vi "1.1)Comandos trigger.vi"() -> ()   [LabVIEW 2014]
panel:
  out "Comando a enviar":string
  in  "?":bool
  out "Comando final":string
  in  "Force":bool
  out "Comandos flanco":string
  out "Comandos pulso":string
  out "Comandos Video":string
  in  "State":bool
  in  "Frecuency":bool
  in  "Mode":u16(ring) items=["Auto", "Normal"]
  in  "Holdoff":dbl(knob) scale=5e-07..10.0
  in  "Nivel":dbl(knob) scale=-20.0..20.0
  out "Tipo de trigger":string
  in  "Opciones de Trigger":enum32{"Flanco", "Video", "Pulso"}(tab)
  in  "Canal":u16(ring) items=["Canal 1", "Canal 2"]
  in  "Slope":u16(ring) items=["Fall", "Rise"]
  in  "Acoplamiento":u16(ring) items=["AC", "DC", "Sin altas frecuencias DC", "Sin bajas frecuencias AC", "Baja sensibilidad DC"]
  in  "Sync":u16(ring) items=["Field", "Line", "Odd", "Even", "LineNum"]
  in  "Polarity":u16(ring) items=["Inverted", "Normal"]
  in  "Lines":dbl(knob) scale=0.0..525.0
  in  "Standard":u16(ring) items=["NTSC", "PAL"]
  in  "Canal":u16(ring) items=["Canal 1", "Canal 2"]
  in  "Width":dbl(knob) scale=3.3e-08..10.0
  in  "When":u16(ring) items=["Equal", "NotEqual", "Inside", "Outside"]
  in  "Polarity":u16(ring) items=["Positivo", "Negativo"]
  in  "Ancho":u16(ring) items=["Polarity", "When", "Width"]
  in  "Canal":u16(ring) items=["Canal 1", "Canal 2"]
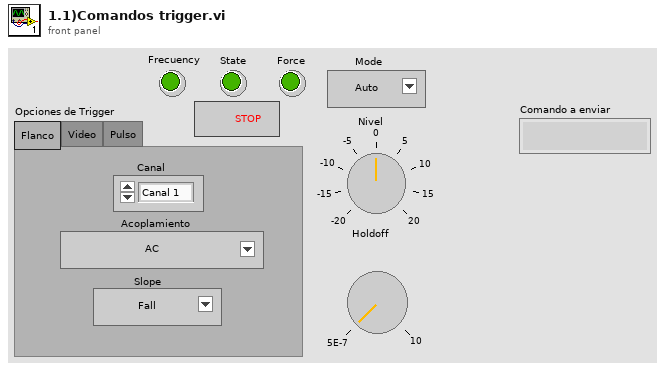
[diagram p1: front panel]
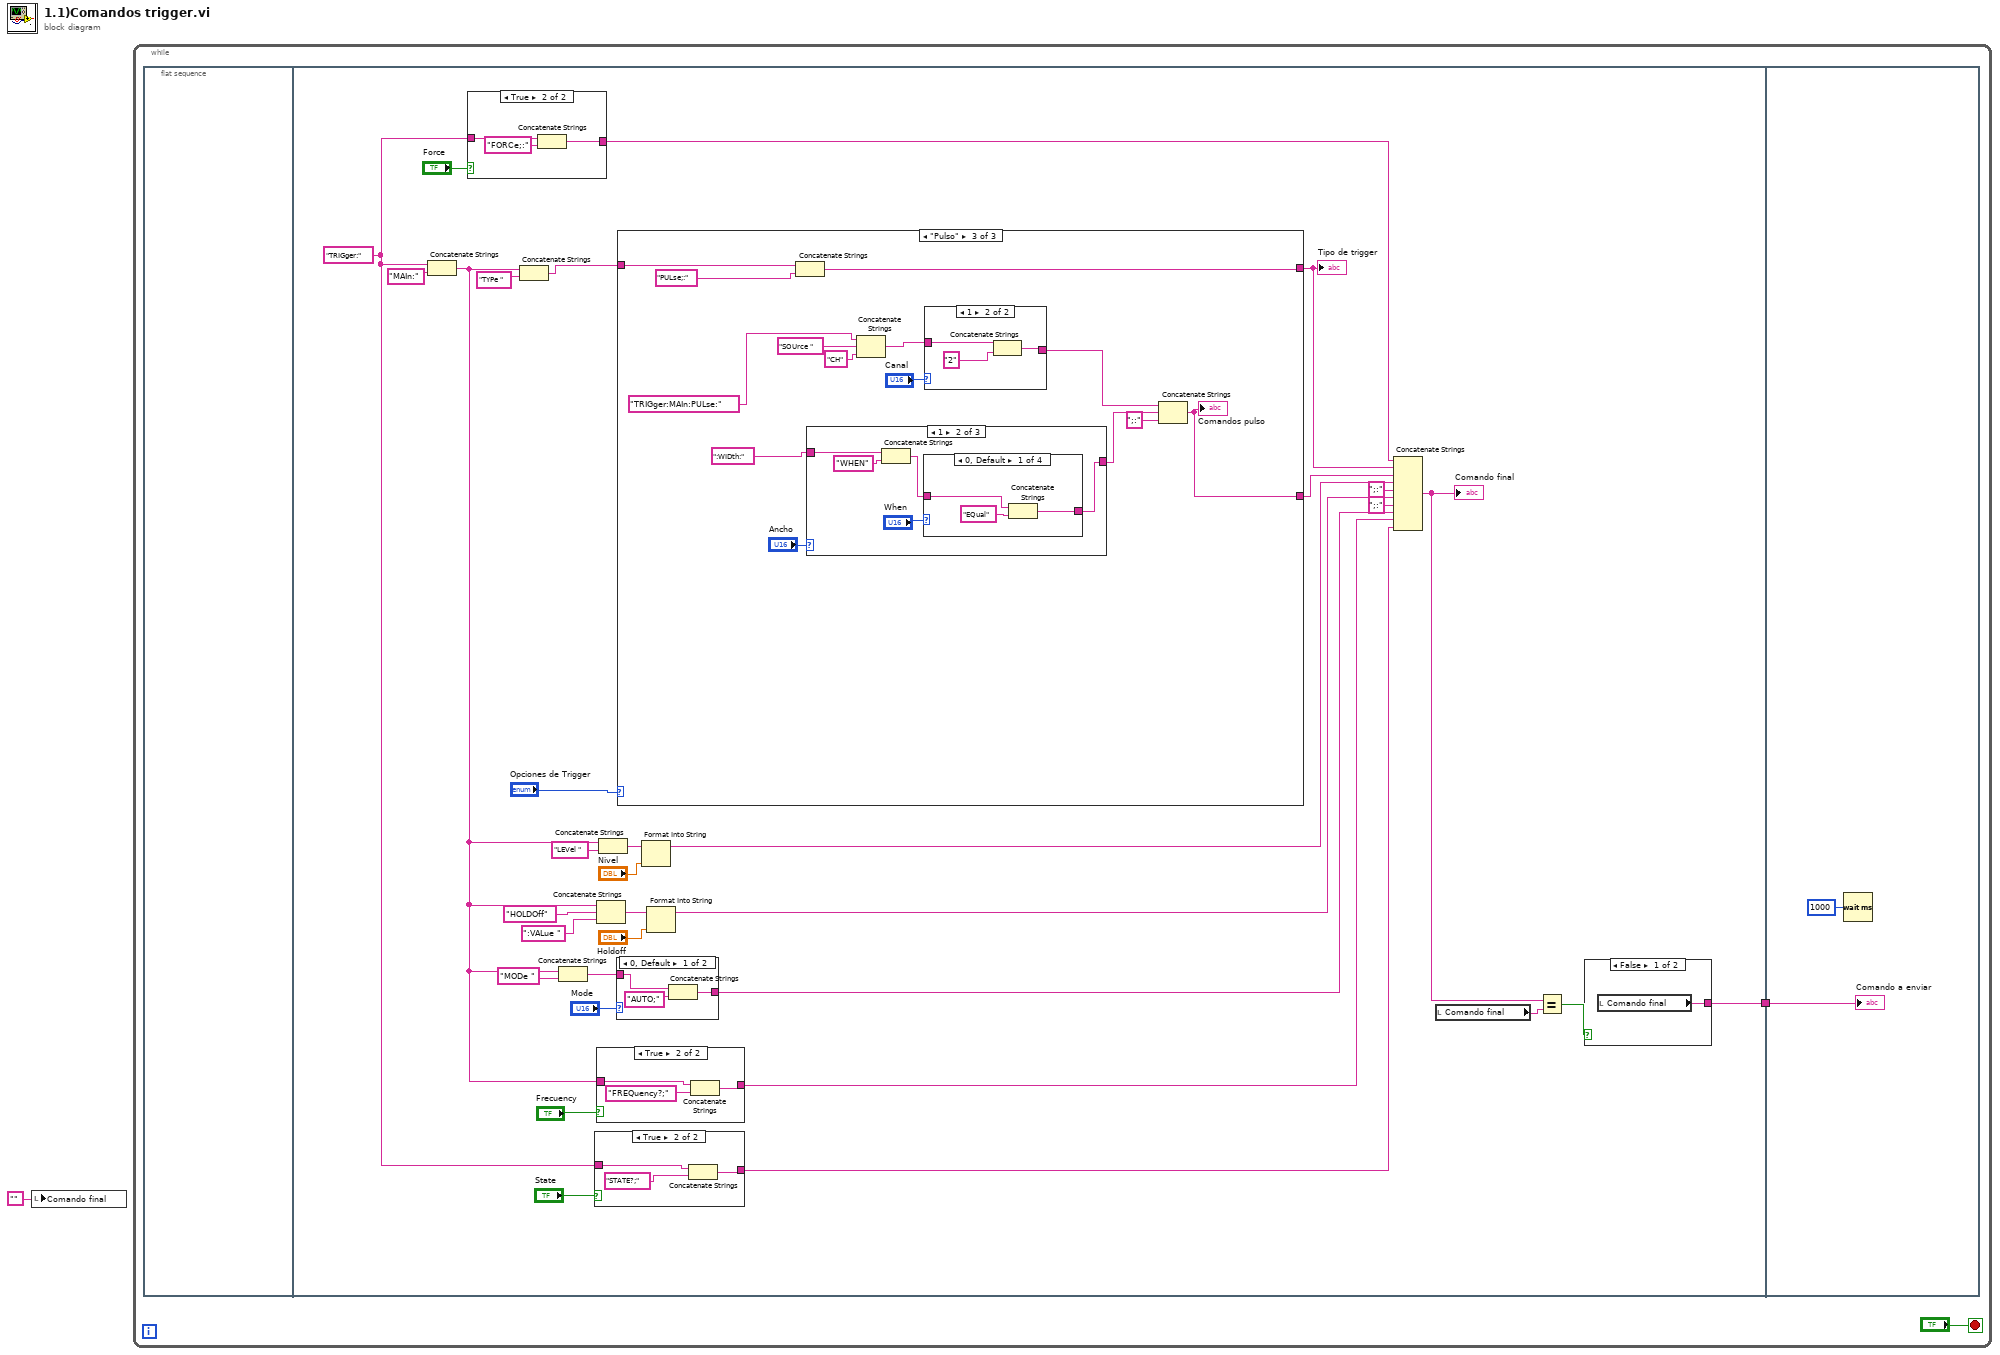
[diagram p0: block diagram]
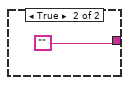
[diagram p2: hidden frame]
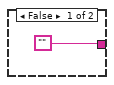
[diagram p3: hidden frame]
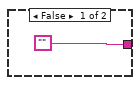
[diagram p4: hidden frame]
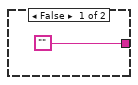
[diagram p5: hidden frame]
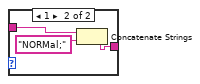
[diagram p6: hidden frame]
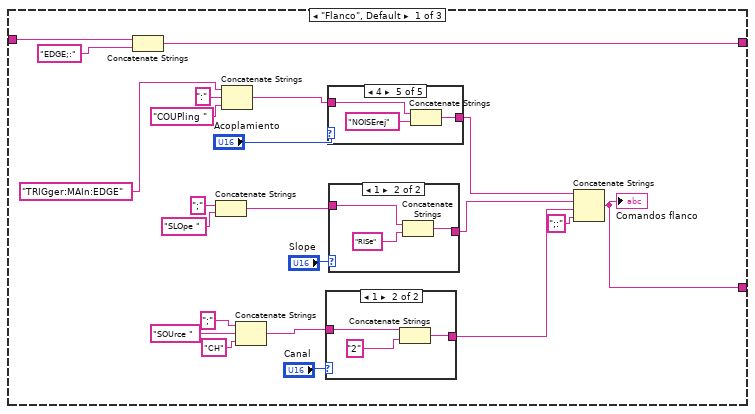
[diagram p7: hidden frame]
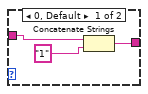
[diagram p8: hidden frame]
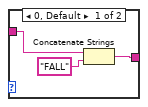
[diagram p9: hidden frame]
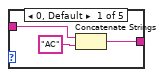
[diagram p10: hidden frame]
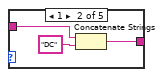
[diagram p11: hidden frame]
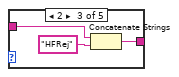
[diagram p12: hidden frame]
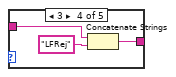
[diagram p13: hidden frame]
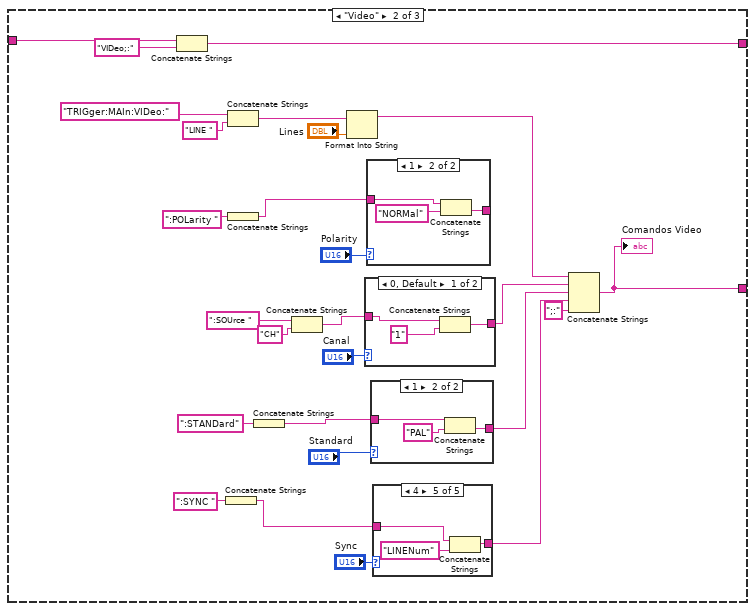
[diagram p14: hidden frame]
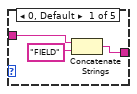
[diagram p15: hidden frame]
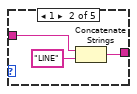
[diagram p16: hidden frame]
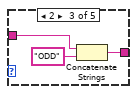
[diagram p17: hidden frame]
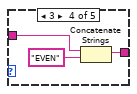
[diagram p18: hidden frame]
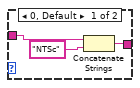
[diagram p19: hidden frame]
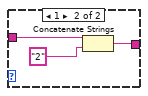
[diagram p20: hidden frame]
diagram:
  n1 = local write "Comando final"("") -> ()
  n2 = while {
    stop <- "?" stop-if-true
    n3 = flat-sequence {
      tunnel: [w6] -> w3
      tunnel: w3 -> [w219]
      frame #0 {
      }
      frame #1 {
        w19 = "TRIGger:"
        n4 = Concatenate Strings(w19, "MAIn:") -> (w20:string)
        n5 = case shown="True" "Force" {
          tunnel: w19 -> [_ w41]
          tunnel: ["" w40] -> w10
          frame False {
          }
          frame True {
            n6 = Concatenate Strings(w41, "FORCe;:") -> (w40:string)
          }
        }
        n7 = Concatenate Strings(w20, "TYPe ") -> (w33:string)
        n8 = Concatenate Strings(w20, "MODe ") -> (w23:string)
        n9 = case shown="True" "State" {
          tunnel: w19 -> [_ w46]
          tunnel: ["" w44] -> w4
          frame False {
          }
          frame True {
            n10 = Concatenate Strings(w46, "STATE?;") -> (w44:string)
          }
        }
        n11 = Concatenate Strings(w20, "HOLDOff", ":VALue ") -> (w27:string)
        n12 = case shown="True" "Frecuency" {
          tunnel: w20 -> [_ w49]
          tunnel: ["" w48] -> w5
          frame False {
          }
          frame True {
            n13 = Concatenate Strings(w49, "FREQuency?;") -> (w48:string)
          }
        }
        n14 = Concatenate Strings(w20, "LEVel ") -> (w31:string)
        n15 = case shown="0, Default" "Mode" {
          tunnel: w23 -> [w53 w56]
          tunnel: [w51 w54] -> w11
          frame 0, Default {
            n16 = Concatenate Strings(w53, "AUTO;") -> (w51:string)
          }
          frame 1 {
            n17 = Concatenate Strings(w56, "NORMal;") -> (w54:string)
          }
        }
        n18 = case shown="\"Pulso\"" "Opciones de Trigger" {
          tunnel: w33 -> [w78 w131 w178]
          tunnel: [w62 w113 w171] -> w17
          tunnel: [w58 w107 w167] -> w16
          frame "Flanco", Default {
            n19 = Concatenate Strings(w78, "EDGE;:") -> (w62:string)
            n20 = Concatenate Strings(";", "SLOpe ") -> (w68:string)
            n21 = Concatenate Strings("TRIGger:MAIn:EDGE", ":", "COUPling ") -> (w74:string)
            n22 = Concatenate Strings(";", "SOUrce ", "CH") -> (w66:string)
            n23 = case shown="1" "Canal" {
              tunnel: w66 -> [w80 w83]
              tunnel: [w79 w82] -> w59
              frame 0, Default {
                n24 = Concatenate Strings(w80, "1") -> (w79:string)
              }
              frame 1 {
                n25 = Concatenate Strings(w83, "2") -> (w82:string)
              }
            }
            n26 = case shown="4" "Acoplamiento" {
              tunnel: w74 -> [w92 w95 w98 w101 w104]
              tunnel: [w91 w94 w97 w100 w103] -> w61
              frame 0, Default {
                n27 = Concatenate Strings(w92, "AC") -> (w91:string)
              }
              frame 1 {
                n28 = Concatenate Strings(w95, "DC") -> (w94:string)
              }
              frame 2 {
                n29 = Concatenate Strings(w98, "HFRej") -> (w97:string)
              }
              frame 3 {
                n30 = Concatenate Strings(w101, "LFRej") -> (w100:string)
              }
              frame 4 {
                n31 = Concatenate Strings(w104, "NOISErej") -> (w103:string)
              }
            }
            n32 = case shown="1" "Slope" {
              tunnel: w68 -> [w86 w89]
              tunnel: [w85 w88] -> w60
              frame 0, Default {
                n33 = Concatenate Strings(w86, "FALL") -> (w85:string)
              }
              frame 1 {
                n34 = Concatenate Strings(w89, "RISe") -> (w88:string)
              }
            }
            n35 = Concatenate Strings(w61, w60, w59, ";:") -> (w58:string)
            "Comandos flanco" <- w58
          }
          frame "Video" {
            n36 = Concatenate Strings(w131, "VIDeo;:") -> (w113:string)
            n37 = Concatenate Strings(":SYNC ") -> (w114:string)
            n38 = Concatenate Strings("TRIGger:MAIn:VIDeo:", "LINE ") -> (w127:string)
            n39 = Concatenate Strings(":POLarity ") -> (w124:string)
            n40 = Concatenate Strings(":STANDard") -> (w117:string)
            n41 = Concatenate Strings(":SOUrce ", "CH") -> (w121:string)
            n42 = Format Into String(initial string=w127, "Lines") -> (resulting string=w111:string)  [unwired: 2 in, 1 out]
            n43 = case shown="0, Default" "Canal" {
              tunnel: w121 -> [w154 w157]
              tunnel: [w153 w156] -> w110
              frame 0, Default {
                n44 = Concatenate Strings(w154, "1") -> (w153:string)
              }
              frame 1 {
                n45 = Concatenate Strings(w157, "2") -> (w156:string)
              }
            }
            n46 = case shown="1" "Polarity" {
              tunnel: w124 -> [w160 w163]
              tunnel: [w159 w162] -> _
              frame 0, Default {
                n47 = Concatenate Strings(w160, "INVERT") -> (w159:string)
              }
              frame 1 {
                n48 = Concatenate Strings(w163, "NORMal") -> (w162:string)
              }
            }
            n49 = case shown="1" "Standard" {
              tunnel: w117 -> [w149 w152]
              tunnel: [w147 w150] -> w109
              frame 0, Default {
                n50 = Concatenate Strings(w149, "NTSc") -> (w147:string)
              }
              frame 1 {
                n51 = Concatenate Strings(w152, "PAL") -> (w150:string)
              }
            }
            n52 = case shown="4" "Sync" {
              tunnel: w114 -> [w133 w136 w139 w142 w145]
              tunnel: [w132 w135 w138 w141 w144] -> w108
              frame 0, Default {
                n53 = Concatenate Strings(w133, "FIELD") -> (w132:string)
              }
              frame 1 {
                n54 = Concatenate Strings(w136, "LINE") -> (w135:string)
              }
              frame 2 {
                n55 = Concatenate Strings(w139, "ODD") -> (w138:string)
              }
              frame 3 {
                n56 = Concatenate Strings(w142, "EVEN") -> (w141:string)
              }
              frame 4 {
                n57 = Concatenate Strings(w145, "LINENum") -> (w144:string)
              }
            }
            n58 = Concatenate Strings(w111, w110, w109, w108, ";:") -> (w107:string)
            "Comandos Video" <- w107
          }
          frame "Pulso" {
            n59 = Concatenate Strings(w178, "PULse;:") -> (w171:string)
            n60 = case shown="1" "Ancho" {
              tunnel: ":WIDth:" -> [w180 w193 w211]
              tunnel: [w179 w190 w207] -> w168
              frame 0, Default {
                n61 = Concatenate Strings(w180, "POLarity ") -> (w181:string)
                n62 = case shown="0, Default" "Polarity" {
                  tunnel: w181 -> [w185 w188]
                  tunnel: [w184 w187] -> w179
                  frame 0, Default {
                    n63 = Concatenate Strings(w185, "POSITIVe") -> (w184:string)
                  }
                  frame 1 {
                    n64 = Concatenate Strings(w188, "NEGAtive") -> (w187:string)
                  }
                }
              }
              frame 1 {
                n65 = Concatenate Strings(w193, "WHEN") -> (w191:string)
                n66 = case shown="0, Default" "When" {
                  tunnel: w191 -> [w196 w199 w202 w205]
                  tunnel: [w195 w198 w201 w204] -> w190
                  frame 0, Default {
                    n67 = Concatenate Strings(w196, "EQual") -> (w195:string)
                  }
                  frame 1 {
                    n68 = Concatenate Strings(w199, "NOTEqual") -> (w198:string)
                  }
                  frame 2 {
                    n69 = Concatenate Strings(w202, "INside") -> (w201:string)
                  }
                  frame 3 {
                    n70 = Concatenate Strings(w205, "OUTside") -> (w204:string)
                  }
                }
              }
              frame 2 {
                n71 = Concatenate Strings(w211, "WIDth ") -> (w209:string)
                n72 = Format Into String(initial string=w209, "Width") -> (resulting string=w207:string)  [unwired: 2 in, 1 out]
              }
            }
            n73 = Concatenate Strings("TRIGger:MAIn:PULse:", "SOUrce ", "CH") -> (w174:string)
            n74 = case shown="1" "Canal" {
              tunnel: w174 -> [w213 w216]
              tunnel: [w212 w215] -> w169
              frame 0, Default {
                n75 = Concatenate Strings(w213, "1") -> (w212:string)
              }
              frame 1 {
                n76 = Concatenate Strings(w216, "2") -> (w215:string)
              }
            }
            n77 = Concatenate Strings(w169, w168, ";:") -> (w167:string)
            "Comandos pulso" <- w167
          }
        }
        "Tipo de trigger" <- w17
        n78 = Format Into String(initial string=w31, "Nivel") -> (resulting string=w15:string)  [unwired: 2 in, 1 out]
        n79 = Format Into String(initial string=w27, "Holdoff") -> (resulting string=w13:string)  [unwired: 2 in, 1 out]
        n80 = Concatenate Strings(w10, w17, w16, w15, ";:", w13, ";:", w11, w5, w4) -> (w9:string)
        "Comando final" <- w9
        n81 = local read "Comando final"() -> (w8:string)
        n82 = Equal?(x=w9, y=w8) -> (x = y?=w7:bool)
        n83 = case shown="False" w7 {
          tunnel: [w37 ""] -> w6
          frame False {
            n84 = local read "Comando final"() -> (w37:string)
          }
          frame True {
          }
        }
      }
      frame #2 {
        n85 = Wait (ms)(milliseconds to wait=u32 1000) -> ()  [unwired: 1 out]
        "Comando a enviar" <- w219
      }
    }
  }
